vi "Launch Downstream Handler.vi"(8 "error in (no error)":errorcluster, 10 "DownStreamMsgHandler":refnum<class "DownStreamMsgHandler.lvclass">, 11 "ServiceManager in":refnum<class "ServiceManager.lvclass">) -> (0 "error out":errorcluster, 3 "ServiceManager out":refnum<class "ServiceManager.lvclass">)   [LabVIEW 2020, in "ServiceManager.lvlib" / "ServiceManager.lvclass"]
uses:
  ServiceManager.lvclass
  DownstreamMsg/DownStreamMsgHandler.lvclass
  <vilib>/ActorFramework/Actor/Actor.lvclass
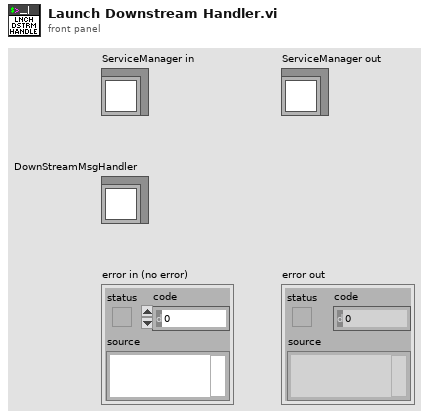
[diagram p1: front panel]
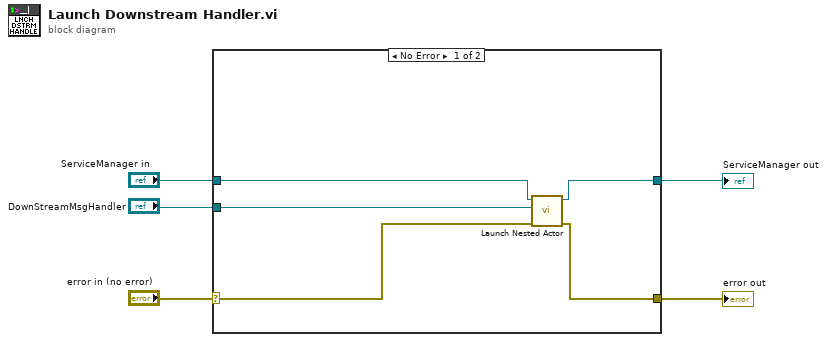
[diagram p0: block diagram]
diagram:
  n1 = case shown="No Error" "error in (no error)" {
    selector: "error in (no error)" -> [w8 w12]
    tunnel: [w6 w12] -> w4
    tunnel: [w9 w11] -> w2
    tunnel: "ServiceManager in" -> [w10 w11]
    tunnel: "DownStreamMsgHandler" -> [w7 _]
    frame No Error {
      n2 = call <vilib>:"Launch Nested Actor.vi"("error in (no error)"=w8, "Nested Actor"=w7, "Caller Actor in"=w10) -> ("error out"=w6:errorcluster, "Caller Actor out"=w9:refnum<class "ServiceManager.lvclass">)  [unwired: 6 in, 1 out]
    }
    frame Error {
    }
  }
  "error out" <- w4
  "ServiceManager out" <- w2
